vi "(SUBVI) - Force Sensor.vi"(10 "Port (Port 1)":T1 items=["Port 1", "Port 2", "Port 3", "Port 4"], 11 "NXT/EV3 2":T2) -> (1 "Raw Value":i16, 2 "Scaled Value":i16, 3 "NXT/EV3":T2)   [LabVIEW 2016]
uses:
  <vilib>/NXT/Subs/LVHSConnector.ctl
  <vilib>/NXT/LegoClasses/BrickReference/BrickReference.lvclass
  <vilib>/NXT/Block Support/NXT_InputPort.ctl
  <vilib>/NXT/Vernier Sensors/Vernier Read/Vernier Sensor NXT_Force10N.vi
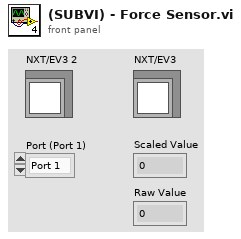
[diagram p1: front panel]
types:
  T1 = typedef "NXT_InputPort.ctl" = u32
  T2 = typedef "LVHSConnector.ctl" = refnum<class "BrickReference.lvclass">
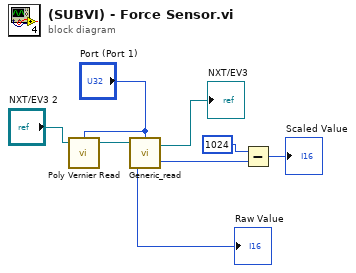
[diagram p0: block diagram]
diagram:
  n1 = call-poly <vilib>:"Poly Vernier Read.vi"("NXT"="NXT/EV3 2", "Port"="Port (Port 1)") -> ("NXT"=w3:T2)  [unwired: 1 in, 2 out]
  n2 = call <vilib>:"Generic_read.vi"("NXT/EV3"=w3, "Port (Port 3)"="Port (Port 1)") -> ("Raw"=→"Raw Value":i16, "Scaled Value"=w6:i16, "NXT/EV3"=→"NXT/EV3":T2)
  n3 = Subtract(x=i16 1024, y=w6) -> (x-y=→"Scaled Value":i16)
